vi "RSZVB Get Trace Unit.vi"(8 "error in (no error)":errorcluster {"code" format="%.0x"}, 9 "Channel (1)":i32=1, 11 "VISA session":refnum<visa-resource-name>) -> (0 "error out":errorcluster {"code" format="%.0x"}, 2 "Format":i32, 3 "dup VISA session":refnum<visa-resource-name>)   [LabVIEW 2011]
doc: "This VI returns the physical unit of the displayed trace.\n\nRemote-control command(s):\nCALCulate<Chn>:FORMat:WQUType?"
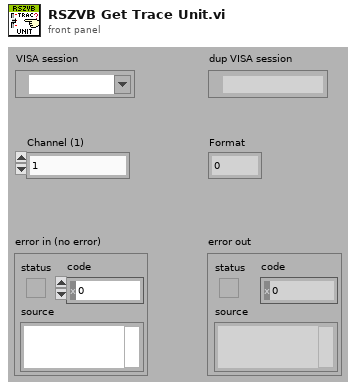
[diagram p1: front panel]
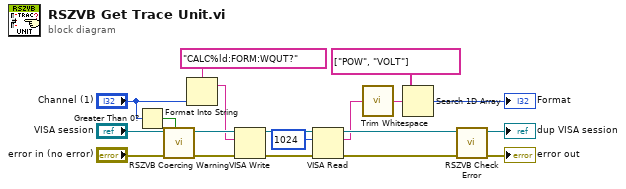
[diagram p0: block diagram]
diagram:
  n1 = Greater Than 0?(x="Channel (1)") -> (x > 0?=w9:bool)
  n2 = call "RSZVB Coercing Warning.vi"("In Range?"=w9, "error in (no error)"="error in (no error)", "VISA session"="VISA session") -> ("error out"=w17:errorcluster, "dup VISA session"=w18:refnum<visa-resource-name>)  [unwired: 7 in]
  n3 = Format Into String(format string="CALC%ld:FORM:WQUT?", "Channel (1)") -> (resulting string=w16:string)  [unwired: 2 in, 1 out]
  n4 = VISA Write(VISA resource name=w18, write buffer=w16, error in (no error)=w17) -> (VISA resource name out=w12:refnum<visa-resource-name>, error out=w13:errorcluster)  [unwired: 1 out]
  n5 = VISA Read(VISA resource name=w12, byte count=u32 1024, error in (no error)=w13) -> (VISA resource name out=w6:refnum<visa-resource-name>, read buffer=w3:string, error out=w5:errorcluster)  [unwired: 1 out]
  n6 = call <vilib>:"Trim Whitespace.vi"("string"=w3) -> ("trimmed string"=w4:string)  [unwired: 1 in]
  n7 = Search 1D Array(1D array=string[] ["POW", "VOLT"], element=w4) -> (index of element=→"Format":i32)  [unwired: 1 in]
  n8 = call "RSZVB Check Error.vi"("error in (no error)"=w5, "VISA session"=w6) -> ("error out"=→"error out":errorcluster, "dup VISA session"=→"dup VISA session":refnum<visa-resource-name>)  [unwired: 8 in]
